vi "Query Marker.vi"(8 "error in (no error)":errorcluster, 10 "Marker Number (1)":u32=1 min=1, 11 "MXA in":refnum<class "MXA.lvclass">) -> (0 "error out":errorcluster, 1 "Marker Level":dbl, 2 "Marker Frequency/Time":dbl, 3 "MXA out":refnum<class "MXA.lvclass">)   [LabVIEW 2020, in "MXA.lvclass"]
uses:
  MXA.lvclass
  C:/Sandbox/RF Bench/Source Code/WiSpry Test Framework/Instruments/Instrument.lvclass
  Instrument.lvclass/Instrument.ctl
  Instrument.lvclass
  <instrlib>/Agilent MXA Series/Agilent MXA Series.lvlib
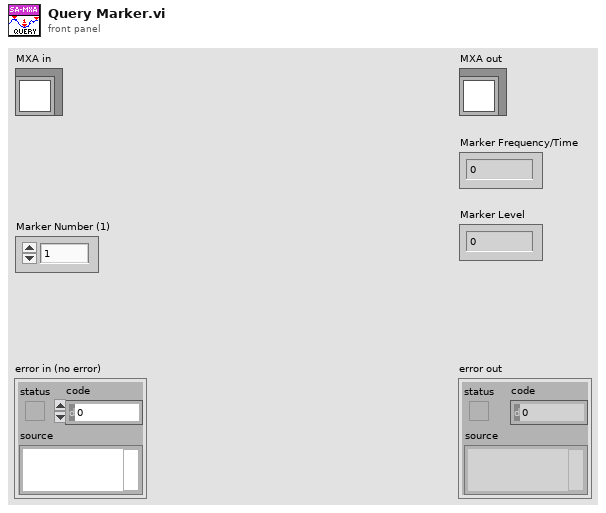
[diagram p1: front panel]
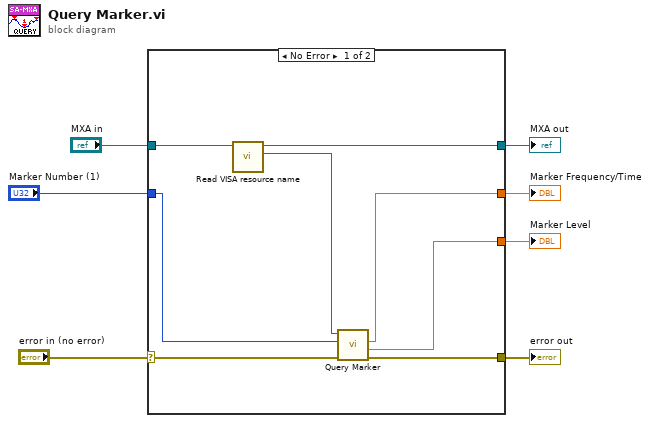
[diagram p0: block diagram]
diagram:
  n1 = case shown="No Error" "error in (no error)" {
    selector: "error in (no error)" -> [w11 w17]
    tunnel: "MXA in" -> [w15 w16]
    tunnel: [w10 w17] -> w5
    tunnel: [w14 w16] -> w6
    tunnel: "Marker Number (1)" -> [w12 _]
    tunnel: [w9 _] -> w2
    tunnel: [w8 _] -> w1
    frame No Error {
      n2 = call "Read VISA resource name.vi"("Instrument in"=w15) -> ("VISA resource name"=w13:refnum<visa-resource-name>, "Instrument out"=w14:refnum<class "MXA.lvclass">)  [unwired: 9 in]
      n3 = call <instrlib>:"Query Marker.vi"("error in (no error)"=w11, "Active Marker (1: Marker1)"=w12, "VISA resource name"=w13) -> ("error out"=w10:errorcluster, "Marker Amplitude"=w9:dbl, "Marker Position"=w8:dbl)  [unwired: 5 in, 1 out]
    }
    frame Error {
    }
  }
  "error out" <- w5
  "MXA out" <- w6
  "Marker Level" <- w2
  "Marker Frequency/Time" <- w1
